vi "Read ERD Dryer.vi"(0 "GEA Inputs":T1 {"Destination" format="%.0x"; "Source" format="%.0x"}, 1 "Read Timeout (ms)":u32=500, 2 "Device Selected":i32, 5 "Retry Count":i32=5, 6 "Read ERD List":T2[](array[typedef]) {"ERD Number" format="%.0x"}, 9 "GEA2 Reference In":refnum<k24>, 11 "Error In":errorcluster, 12 "Standalone?":bool, 13 "Verify ERD Response?":bool) -> (4 "Data Returned":string, 7 "ERD Data Out":T4[](array[typedef]) {"ERD Number" format="%.0x"}, 10 "GEA2 Reference Out":refnum<k24>, 15 "Error Out":errorcluster)   [LabVIEW 2014]
doc: "This standalone VI reads the next message on the GEA2 bus OR waits until it receives a message with the command or data you specify. (.* = anything)"
uses:
  Common/LabVIEW GEA2 Toolkit/LabVIEW_GEA2_Toolkit.lvlibp/type defs/ERD Read Data Out.ctl
  Common/LabVIEW GEA2 Toolkit/LabVIEW_GEA2_Toolkit.lvlibp/type defs/ERD Read Data In.ctl
  Common/LabVIEW GEA2 Toolkit/LabVIEW_GEA2_Toolkit.lvlibp/type defs/Data Type.ctl
  Common/LabVIEW GEA2 Toolkit/LabVIEW_GEA2_Toolkit.lvlibp/type defs/Source_Destination.ctl
  C:/Automation/DLLs/PC Dot Net/GeaCommunication.dll
  Common/LabVIEW GEA2 Toolkit/LabVIEW_GEA2_Toolkit.lvlibp
  C:/Automation/DLLs/PC Tools .NET/GeaCommunication.dll
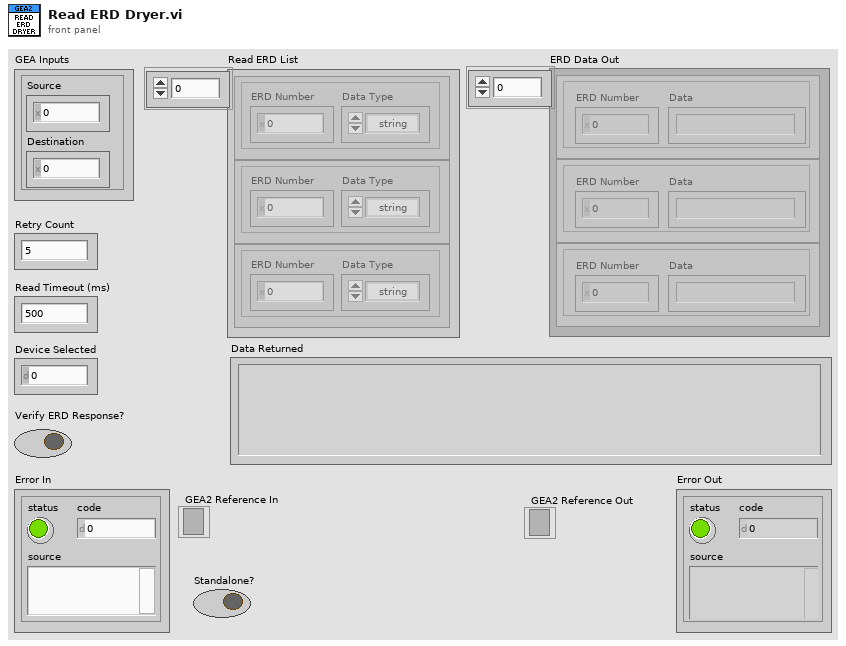
[diagram p1: front panel]
types:
  T1 = typedef "LabVIEW_GEA2_Toolkit.lvlibp/Source_Destination.ctl" = cluster{"Source":u8, "Destination":u8}
  T2 = typedef "LabVIEW_GEA2_Toolkit.lvlibp/ERD Read Data In.ctl" = cluster{"ERD Number":u16, "Data Type":T3}
  T3 = typedef "LabVIEW_GEA2_Toolkit.lvlibp/Data Type.ctl" = enum16{"string", "boolean", "uint8_t", "uint16_t", "uint32_t", "uint64_t", "int8_t", "int16_t", "int32_t", "int64_t"}
  T4 = typedef "LabVIEW_GEA2_Toolkit.lvlibp/ERD Read Data Out.ctl" = cluster{"ERD Number":u16, "Data":string}
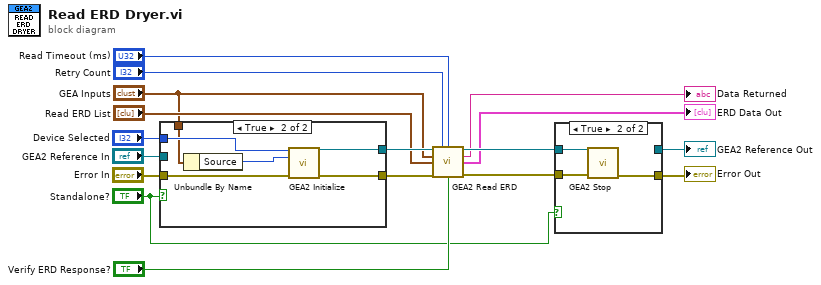
[diagram p0: block diagram]
diagram:
  n1 = case shown="True" "Standalone?" {
    tunnel: [w19 w25] -> w15
    tunnel: "Error In" -> [w19 w24]
    tunnel: "Device Selected" -> [_ w23]
    tunnel: [w18 w22] -> w7
    tunnel: "GEA Inputs" -> [_ w21]
    tunnel: "GEA2 Reference In" -> [w18 _]
    frame False {
    }
    frame True {
      n2 = Unbundle By Name(w21) -> ("Source"=w20:u8)
      n3 = call "GEA2 Initialize.vi"("Board Index"=w23, "Source Address"=w20, "error in"=w24) -> ("GEA2 Reference Out"=w22:refnum<k24>, "error out"=w25:errorcluster)  [unwired: 10 in, 1 out]
    }
  }
  n4 = call "GEA2 Read ERD.vi"("GEA2 Reference In"=w7, "Retry Count"="Retry Count", "Read Timeout (ms)"="Read Timeout (ms)", "GEA Inputs"="GEA Inputs", "Read ERD List"="Read ERD List", "Error In"=w15, "Verify ERD Response?"="Verify ERD Response?") -> ("GEA2 Reference Out"=w16:refnum<k24>, "Raw Data Out"=→"Data Returned":string, "ERD Data Out"=→"ERD Data Out":T4[], "Error Out"=w17:errorcluster)  [unwired: 5 in]
  n5 = case shown="True" "Standalone?" {
    tunnel: w17 -> [w26 w30]
    tunnel: w16 -> [w27 w29]
    tunnel: [w26 w28] -> w13
    tunnel: [w27 _] -> w1
    frame False {
    }
    frame True {
      n6 = call "GEA2 Stop.vi"("GEA2 Reference In"=w29, "Error In"=w30) -> ("Error Out"=w28:errorcluster)  [unwired: 13 in]
    }
  }
  "Error Out" <- w13
  "GEA2 Reference Out" <- w1
